vi "parse_header-multiple.vi"(8 "error in (no error)":errorcluster, 10 "header_to_get []":string[](array[string]), 11 "headers":string) -> (0 "error out":errorcluster, 3 "header []":cluster{"header":string, "value":string}[](array[cluster]))   [LabVIEW 2015, in "lv-dropbox.lvlib"]
uses:
  lv-dropbox.lvlib
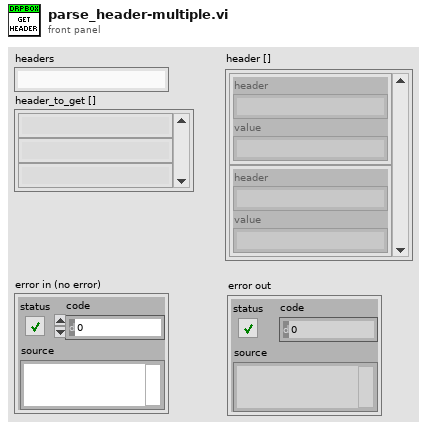
[diagram p1: front panel]
types:
  T1 = cluster{"header_to_get []":string, "trimmed string":string}
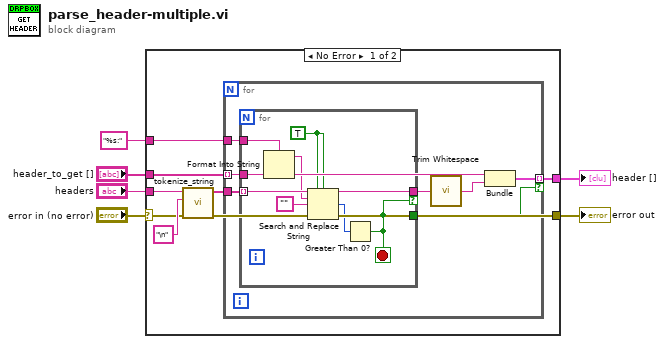
[diagram p0: block diagram]
diagram:
  n1 = case shown="No Error" "error in (no error)" {
    selector: "error in (no error)" -> [w12 w31]
    tunnel: [w10 w31] -> w1
    tunnel: "headers" -> [w14 _]
    tunnel: "header_to_get []" -> [w9 _]
    tunnel: "%s:" -> [w8 _]
    tunnel: [w7 _] -> w2
    frame No Error {
      n2 = call "tokenize_string.vi"("error in (no error)"=w12, "delimiter"="\n", "input_string"=w14) -> ("error out"=w10:errorcluster, "delimited_string []"=w11:string[])  [unwired: 5 in, 2 out]
      n3 = for {
        tunnel: w11 -> [w21]
        tunnel: w9 -> [w18] mode=indexing
        tunnel: w8 -> [w20]
        tunnel: [w16] -> w7 mode=indexing if=w15
        n4 = for {
          tunnel: w21 -> [w28] mode=indexing
          tunnel: w18 -> [w29]
          tunnel: w20 -> [w30]
          tunnel: [w23] -> w19 if=w22
          tunnel: [w22] -> w15
          stop <- w22 stop-if-true
          w27 = TRUE ("replace all? (F)")
          n5 = Format Into String(format string=w30, w29) -> (resulting string=w26:string)  [unwired: 2 in, 1 out]
          n6 = Search and Replace String(replace all?=w27, case sensitive?=w27, input string=w28, search string=w26, replace string="") -> (result string=w23:string, number of replacements=w24:i32)  [unwired: 3 in, 2 out]
          n7 = Greater Than 0?(x=w24) -> (x > 0?=w22:bool)
        }
        n8 = call <vilib>:"Trim Whitespace.vi"("string"=w19) -> ("trimmed string"=w17:string)  [unwired: 1 in]
        n9 = Bundle("header_to_get []"=w18, "trimmed string"=w17) -> (w16:T1)  [unwired: 1 in]
      }
    }
    frame Error {
    }
  }
  "header []" <- w2
  "error out" <- w1
